vi "AVI playback timing control.vi"(7 "Disable PID? (T)":bool=TRUE, 9 "integral time (Ti, min)":dbl=0.01 min=0.0 max=2142532154361346.0 step=0.01 format="%#_13g", 11 "proportional gain (Kc)":dbl=0.7 min=0.0 step=0.05 format="%#_13g") -> (0 "Frame period set-point (ms)":dbl, 1 "Actual frame rate (fps)":dbl format="Actual frame rate %#_g (fps)", 2 "Frame rate set OR original (fps)":dbl format="Frame rate set %#_g (fps)", 3 "Original frame rate (fps)":dbl format="Original frame rate %#_g (fps)")   [LabVIEW 2020]
panel:
  out "Original frame period (ms)":i32
  out "Loop time (ms)":u32
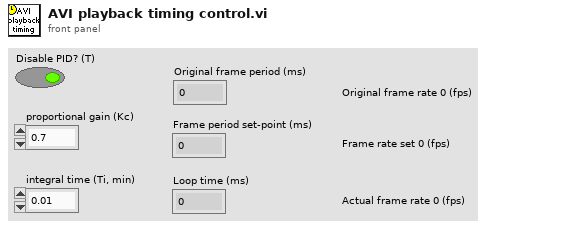
[diagram p1: front panel]
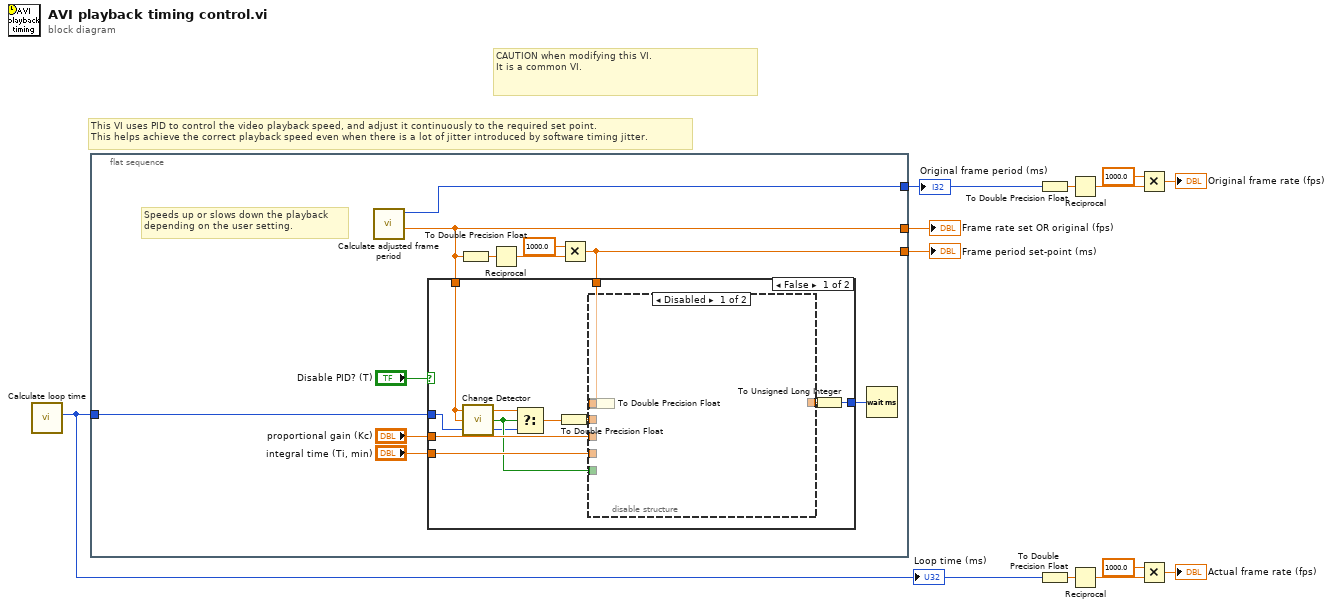
[diagram p0: block diagram]
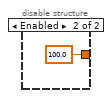
[diagram p2: hidden frame]
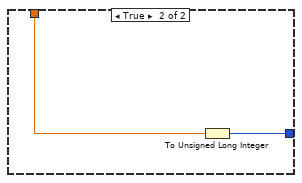
[diagram p3: hidden frame]
diagram:
  # "CAUTION when modifying this VI.\nIt is a common VI."
  # "This VI uses PID to control the video playback speed, and adjust it continuously to the required set point.\nThis helps achieve the correct playback speed even when there is a lot of jitter introduced by software timing jitter."
  n1 = call <userlib>:"Calculate loop time.vi"() -> ("Loop time (ms)"=w3:u32)  [unwired: 11 in]
  "Loop time (ms)" <- w3
  n2 = flat-sequence {
    tunnel: w3 -> [w20]
    tunnel: [w14] -> w2
    tunnel: [w18] -> w4
    tunnel: [w13] -> w1
    frame #0 {
      # "Speeds up or slows down the playback\ndepending on the user setting."
      n3 = call "Calculate adjusted frame period.vi"() -> ("Frame rate set OR original (fps)"=w14:dbl, "Original frame period (ms)"=w18:i32)  [unwired: 9 in, 1 out]
      n4 = To Double Precision Float(number=w14) -> (double precision float=w15:dbl)
      n5 = Reciprocal(x=w15) -> (1/x=w16:dbl)
      n6 = Multiply(x=1000.0, y=w16) -> (x*y=w13:dbl)
      n7 = case shown="False" "Disable PID? (T)" {
        tunnel: "proportional gain (Kc)" -> [w32 _]
        tunnel: "integral time (Ti, min)" -> [w31 _]
        tunnel: [w30 w36] -> w21
        tunnel: w14 -> [w27 _]
        tunnel: w20 -> [w26 _]
        tunnel: w13 -> [w24 w37]
        frame False {
          n8 = call <userlib>:"Change Detector.vi"("Value"=w27) -> ("Changed?"=w28:bool)
          n9 = Select(t=w27, s=w28, f=w26) -> (s? t:f=w25:dbl)
          n10 = To Double Precision Float(number=w25) -> (double precision float=w29:dbl)
          n11 = disable-structure shown="Disabled" {
            disable-tunnel: [_ 100.0 ("output")] -> w33
            disable-tunnel: w32 -> [_ _]
            disable-tunnel: w31 -> [_ _]
            disable-tunnel: w29 -> [_ _]
            disable-tunnel: w28 -> [_ _]
            disable-tunnel: w24 -> [w34 _]
            frame Disabled {
              n12 = To Double Precision Float(number=w34) -> ()  [unwired: 1 out]
            }
            frame Enabled {
            }
          }
          n13 = To Unsigned Long Integer(number=w33) -> (unsigned 32bit integer=w30:u32)
        }
        frame True {
          n14 = To Unsigned Long Integer(number=w37) -> (unsigned 32bit integer=w36:u32)
        }
      }
      n15 = Wait (ms)(milliseconds to wait=w21) -> ()  [unwired: 1 out]
    }
  }
  n16 = To Double Precision Float(number=w4) -> (double precision float=w5:dbl)
  n17 = To Double Precision Float(number=w3) -> (double precision float=w9:dbl)
  n18 = Reciprocal(x=w5) -> (1/x=w6:dbl)
  n19 = Reciprocal(x=w9) -> (1/x=w10:dbl)
  n20 = Multiply(x=1000.0, y=w6) -> (x*y=→"Original frame rate (fps)":dbl)
  n21 = Multiply(x=1000.0, y=w10) -> (x*y=→"Actual frame rate (fps)":dbl)
  "Frame period set-point (ms)" <- w1
  "Original frame period (ms)" <- w4
  "Frame rate set OR original (fps)" <- w2
